vi "Draw Marker Lines.vi"(6 "Type":T1, 9 "Marker Options":T2={"Color"=16723218, "pen"={"Width"=2, "Style"=enum."Solid"}, "font"={"Font Name"="Arial", "Size"=16, "Strikeout?"=FALSE, "Italic?"=FALSE, "Underline?"=FALSE, "Outline?"=FALSE, "Shadow?"=FALSE, "Bold?"=FALSE, "FontColor"=0}, "caption"=""}, 10 "position":T3, 11 "picture":picture) -> (3 "new picture":picture)   [LabVIEW 2014, in "Graph Extensions.lvlib"]
doc: "Draw the appropriate line for markers, depending on the type"
uses:
  Graph Extensions.lvlib
  <vilib>/Utility/miscctls.llb/LVPoint32TypeDef.ctl
  controls/MarkerOptions.ctl
  controls/markerType.ctl
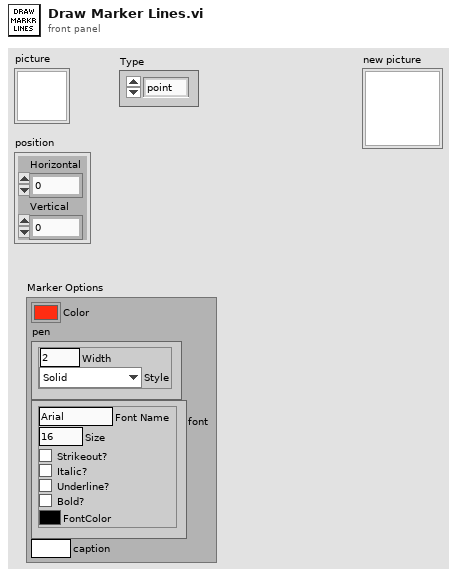
[diagram p1: front panel]
types:
  T1 = typedef "Graph Extensions.lvlib/markerType.ctl" = enum16{"point", "arrow", "horiz", "vert", "vert range", "horiz range", "box"}
  T2 = typedef "Graph Extensions.lvlib/MarkerOptions.ctl" = cluster{"Color":u32, "pen":cluster{"Width":u16, "Style":enum32{"Solid", "Dash", "Dot", "DashDot", "DashDotDot"}}, "font":cluster{"Font Name":string, "Size":i16, "Strikeout?":bool, "Italic?":bool, "Underline?":bool, "Outline?":bool, "Shadow?":bool, "Bold?":bool, "FontColor":u32}, "caption":string}
  T3 = typedef "LVPoint32TypeDef.ctl" = cluster{"Horizontal":i32, "Vertical":i32}
  T4 = enum32{"Solid", "Dash", "Dot", "DashDot", "DashDotDot"}
  T5 = cluster{"Font Name:":string, "Size":i16, "Strikeout?":bool, "Italic?":bool, "Underline?":bool, "Outline?":bool, "Shadow?":bool, "Bold?":bool}
  T6 = enum16{"User-specified Font", "Application Font", "System Font", "Dialog Font"}
  T7 = cluster{"Font Name":string, "Size":i16, "Strikeout?":bool, "Italic?":bool, "Underline?":bool, "Outline?":bool, "Shadow?":bool, "Bold?":bool, "FontColor":u32}
  T8 = cluster{"Width":u16, "Style":enum32{"Solid", "Dash", "Dot", "DashDot", "DashDotDot"}}
  T9 = cluster{"left":i16, "top":i16, "right":i16, "bottom":i16}
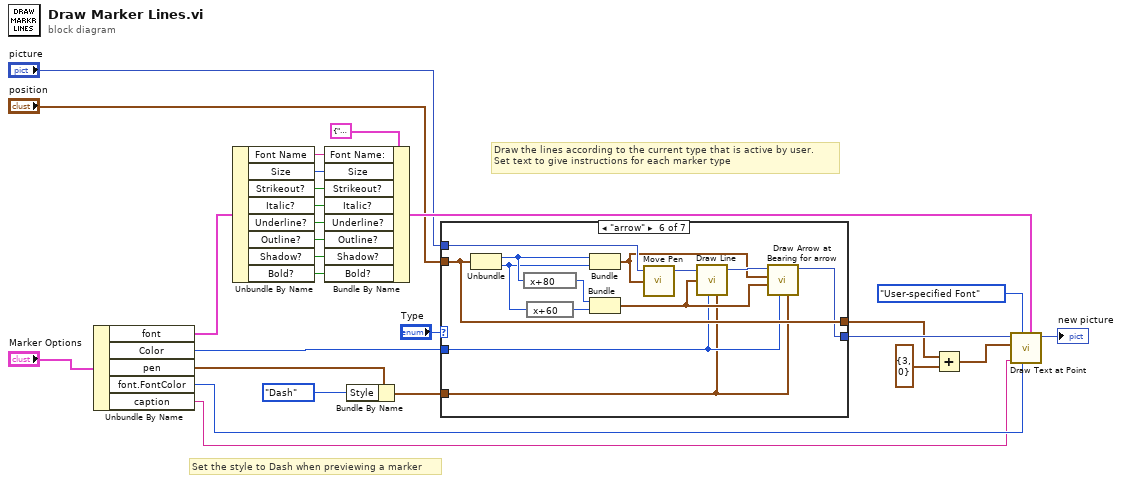
[diagram p0: block diagram]
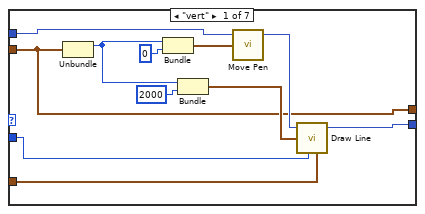
[diagram p2: hidden frame]
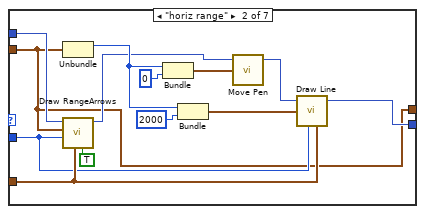
[diagram p3: hidden frame]
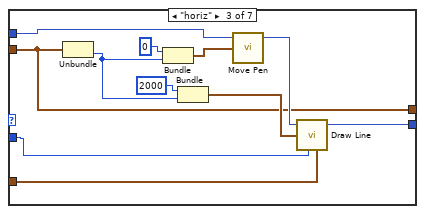
[diagram p4: hidden frame]
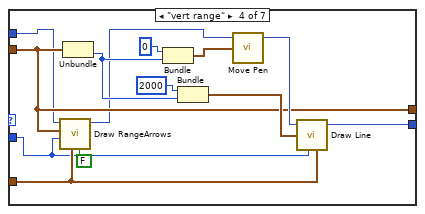
[diagram p5: hidden frame]
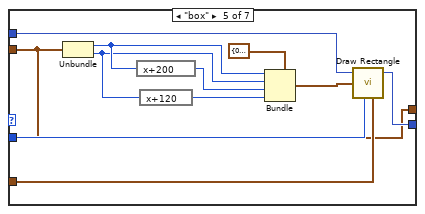
[diagram p6: hidden frame]
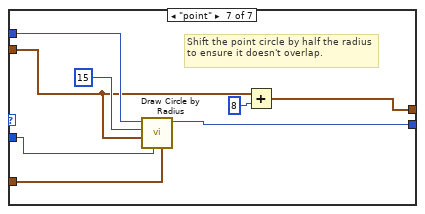
[diagram p7: hidden frame]
diagram:
  # "Set the style to Dash when previewing a marker"
  # "Draw the lines according to the current type that is active by user.\nSet text to give instructions for each marker type"
  n1 = Unbundle By Name("Marker Options") -> ("font"=w4:T7, "Color"=w10:u32, "pen"=w8:T8, "font.FontColor"=w21:u32, "caption"=w1:string)
  n2 = Unbundle By Name(w4) -> ("Font Name"=w19:string, "Size"=w18:i16, "Strikeout?"=w17:bool, "Italic?"=w16:bool, "Underline?"=w15:bool, "Outline?"=w14:bool, "Shadow?"=w13:bool, "Bold?"=w12:bool)
  n3 = Bundle By Name(cluster=T5 {"Font Name:"="", "Size"=12, "Strikeout?"=FALSE, "Italic?"=FALSE, "Underline?"=FALSE, "Outline?"=FALSE, "Shadow?"=FALSE, "Bold?"=FALSE} ("[user-specified font]"), "Font Name:"=w19, "Size"=w18, "Strikeout?"=w17, "Italic?"=w16, "Underline?"=w15, "Outline?"=w14, "Shadow?"=w13, "Bold?"=w12) -> (w11:T5)
  n4 = Bundle By Name(cluster=w8, "Style"=T4."Dash") -> (w7:T8)
  n5 = case shown="\"arrow\"" "Type" {
    tunnel: "position" -> [w28 w40 w55 w65 w76 w99 w102]
    tunnel: [w36 w49 w61 w74 w84 w91 w107] -> w24
    tunnel: "picture" -> [w31 w44 w52 w64 w86 w98 w103]
    tunnel: w10 -> [w30 w41 w54 w66 w85 w89 w106]
    tunnel: w7 -> [w29 w42 w53 w67 w77 w87 w104]
    tunnel: [w28 w40 w55 w65 w76 w99 w100] -> w5
    frame "vert" {
      n6 = Unbundle(w28) -> ("Horizontal"=w38:i32)  [unwired: 1 out]
      n7 = Bundle("Horizontal"=w38, "top"=i16 0) -> (w32:cluster{"Horizontal":i32, "top":i16})  [unwired: 1 in]
      n8 = Bundle("Horizontal"=w38, "top"=i16 2000) -> (w37:cluster{"Horizontal":i32, "top":i16})  [unwired: 1 in]
      n9 = call <vilib>:"Move Pen.vi"("new position"=w32, "picture"=w31) -> ("new picture"=w35:picture)  [unwired: 3 in]
      n10 = call <vilib>:"Draw Line.vi"("picture"=w35, "end point"=w37, "color(black)"=w30, "pen"=w29) -> ("new picture"=w36:picture)  [unwired: 5 in]
    }
    frame "horiz range" {
      n11 = Unbundle(w40) -> ("Horizontal"=w51:i32)  [unwired: 1 out]
      n12 = call "Draw RangeArrows.vi"("Vertical"=TRUE, "pen"=w42, "Color"=w41, "position"=w40, "picture"=w44) -> ("new picture"=w43:picture)  [unwired: 6 in]
      n13 = Bundle("Horizontal"=w51, "top"=i16 0) -> (w45:cluster{"Horizontal":i32, "top":i16})  [unwired: 1 in]
      n14 = Bundle("Horizontal"=w51, "top"=i16 2000) -> (w50:cluster{"Horizontal":i32, "top":i16})  [unwired: 1 in]
      n15 = call <vilib>:"Move Pen.vi"("new position"=w45, "picture"=w43) -> ("new picture"=w48:picture)  [unwired: 3 in]
      n16 = call <vilib>:"Draw Line.vi"("picture"=w48, "end point"=w50, "color(black)"=w41, "pen"=w42) -> ("new picture"=w49:picture)  [unwired: 5 in]
    }
    frame "horiz" {
      n17 = Unbundle(w55) -> ("Vertical"=w57:i32)  [unwired: 1 out]
      n18 = Bundle("top"=i16 0, "Vertical"=w57) -> (w59:cluster{"top":i16, "Vertical":i32})  [unwired: 1 in]
      n19 = Bundle("top"=i16 2000, "Vertical"=w57) -> (w62:cluster{"top":i16, "Vertical":i32})  [unwired: 1 in]
      n20 = call <vilib>:"Move Pen.vi"("new position"=w59, "picture"=w52) -> ("new picture"=w60:picture)  [unwired: 3 in]
      n21 = call <vilib>:"Draw Line.vi"("picture"=w60, "end point"=w62, "color(black)"=w54, "pen"=w53) -> ("new picture"=w61:picture)  [unwired: 5 in]
    }
    frame "vert range" {
      n22 = call "Draw RangeArrows.vi"("Vertical"=FALSE, "pen"=w67, "Color"=w66, "position"=w65, "picture"=w64) -> ("new picture"=w63:picture)  [unwired: 6 in]
      n23 = Unbundle(w65) -> ("Vertical"=w70:i32)  [unwired: 1 out]
      n24 = Bundle("top"=i16 0, "Vertical"=w70) -> (w72:cluster{"top":i16, "Vertical":i32})  [unwired: 1 in]
      n25 = Bundle("top"=i16 2000, "Vertical"=w70) -> (w75:cluster{"top":i16, "Vertical":i32})  [unwired: 1 in]
      n26 = call <vilib>:"Move Pen.vi"("new position"=w72, "picture"=w63) -> ("new picture"=w73:picture)  [unwired: 3 in]
      n27 = call <vilib>:"Draw Line.vi"("picture"=w73, "end point"=w75, "color(black)"=w66, "pen"=w67) -> ("new picture"=w74:picture)  [unwired: 5 in]
    }
    frame "box" {
      n28 = Unbundle(w76) -> ("Horizontal"=w82:i32, "Vertical"=w79:i32)
      n29 = expression code="x+200"(w82) -> (w81:i32)
      n30 = expression code="x+120"(w79) -> (w78:i32)
      n31 = Bundle(cluster=T9 {"left"=0, "top"=0, "right"=0, "bottom"=0} ("rect"), "left"=w82, "top"=w79, "right"=w81, "bottom"=w78) -> (w83:T9)
      n32 = call <vilib>:"Draw Rectangle.vi"("picture"=w86, "rect"=w83, "color(black)"=w85, "pen"=w77) -> ("new picture"=w84:picture)  [unwired: 5 in]
    }
    frame "arrow" {
      n33 = Unbundle(w99) -> ("Horizontal"=w93:i32, "Vertical"=w92:i32)
      n34 = expression code="x+80"(w93) -> (w95:i32)
      n35 = expression code="x+60"(w92) -> (w94:i32)
      n36 = Bundle("Horizontal"=w93, "Vertical"=w92) -> (w88:cluster{"Horizontal":i32, "Vertical":i32})  [unwired: 1 in]
      n37 = Bundle("Horizontal"=w95, "Vertical"=w94) -> (w90:cluster{"Horizontal":i32, "Vertical":i32})  [unwired: 1 in]
      n38 = call <vilib>:"Move Pen.vi"("new position"=w88, "picture"=w98) -> ("new picture"=w97:picture)  [unwired: 3 in]
      n39 = call <vilib>:"Draw Line.vi"("picture"=w97, "end point"=w90, "color(black)"=w89, "pen"=w87) -> ("new picture"=w96:picture)  [unwired: 5 in]
      n40 = call "Draw Arrow at Bearing for arrow.vi"("pen"=w87, "color(black)"=w89, "P2"=w90, "P1"=w88, "new picture in"=w96) -> ("new picture out"=w91:picture)  [unwired: 6 in]
    }
    frame "point" {
      # "Shift the point circle by half the radius to ensure it doesn't overlap."
      n41 = call <vilib>:"Draw Circle by Radius.vi"("pen"=w104, "color(black)"=w106, "pixel center"=w102, "radius"=i16 15, "picture"=w103) -> ("new picture"=w107:picture)  [unwired: 6 in]
      n42 = Add(x=w102, y=8 ("Horizontal")) -> (x+y=w100:T3)
    }
  }
  n43 = Add(x=w5, y=T3 {"Horizontal"=3, "Vertical"=0}) -> (x+y=w26:T3)
  n44 = call <vilib>:"Draw Text at Point.vi"("[user-specified font]"=w11, "text color(black)"=w21, "desired font(Application)"=T6."User-specified Font", "text"=w1, "origin"=w26, "picture"=w24) -> ("new picture"=→"new picture":picture)  [unwired: 4 in, 1 out]
